vi "construct.vi"(8 "error in (no error)":errorcluster, 9 "configuration name":string, 10 "load config file?":bool=TRUE, 11 "ExperimentControllerDL090130Interval in":refnum<class "ExperimentControllerDL090130Interval.lvclass">) -> (0 "error out":errorcluster, 3 "ExperimentControllerDL090130Interval out":refnum<class "ExperimentControllerDL090130Interval.lvclass">)   [LabVIEW 2010, in "ExperimentControllerDL090130Interval.lvclass"]
uses:
  ExperimentControllerDL090130Interval.lvclass
  GenericExperimentController/GenericExperimentController/GenericExperimentController.lvclass
  ExperimentControllerDL090130Interval.lvclass/ExperimentControllerDL090130Interval.ctl
  Sweep/GenericSweep/GenericSweep/GenericSweep.lvclass
  common/classes/ErrorController/ErrorController/class_data.vi
  common/classes/GenericComponent/GenericComponent/GenericComponent.lvclass
  common/classes/ErrorController/ErrorController/ErrorController.lvclass
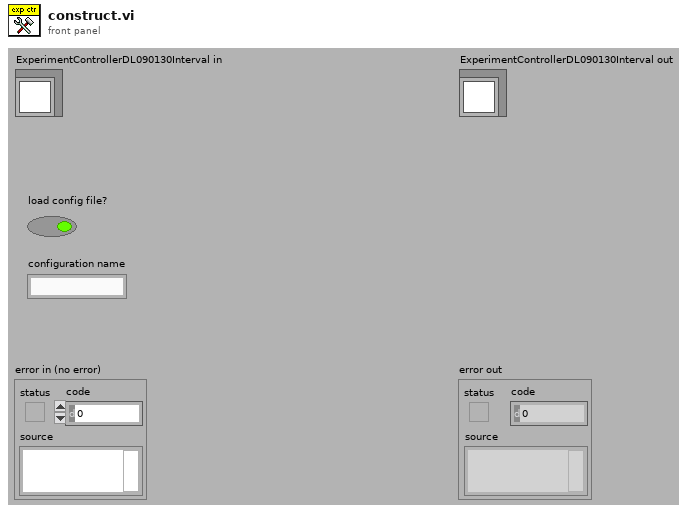
[diagram p1: front panel]
types:
  T1 = typedef "plugin_specification.ctl" = cluster{"class path":string, "configuration":string, "label":string, "settings name":string}
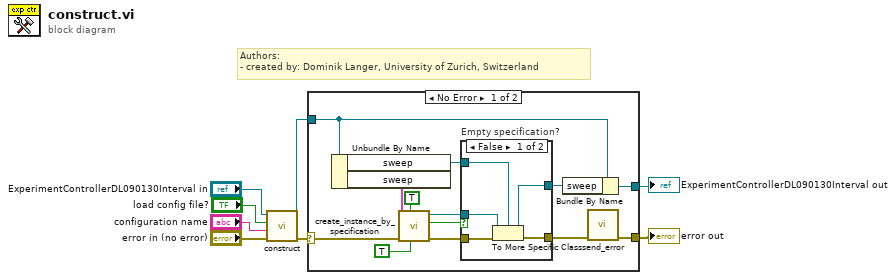
[diagram p0: block diagram]
diagram:
  # "Authors: \n- created by: Dominik Langer, University of Zurich, Switzerland"
  n1 = call-parent "construct.vi"("error in (no error)"="error in (no error)", "configuration name"="configuration name", "load config file?"="load config file?", "GenericPlugin in"="ExperimentControllerDL090130Interval in") -> ("error out"=w4:errorcluster, "GenericPlugin out"=w3:refnum<class "ExperimentControllerDL090130Interval.lvclass">)  [unwired: 6 in]
  n2 = case shown="No Error" w4 {
    selector: w4 -> [w18 w29]
    tunnel: w3 -> [w20 w28]
    tunnel: [w11 w29] -> w2
    tunnel: [w19 w28] -> w1
    frame No Error {
      n3 = Unbundle By Name(w20) -> ("sweep"=w21:refnum<class "GenericSweep.lvclass">, "sweep"=w17:T1)
      n4 = call "create_instance_by_specification.vi"("be tolerant against empty specification?"=TRUE, "call constructor?"=TRUE, "error in (no error)"=w18, "component specification"=w17) -> ("error out"=w16:errorcluster, "empty specification!"=w9:bool, "GenericPlugin out"=w13:refnum<class "GenericComponent.lvclass">)  [unwired: 5 in]
      n5 = case "Empty specification?" shown="False" w9 {
        tunnel: w21 -> [w26 _]
        tunnel: w16 -> [w25 w27]
        tunnel: [w24 _] -> w15
        tunnel: w13 -> [w23 _]
        tunnel: [w22 w27] -> w12
        frame False {
          n6 = To More Specific Class(target class=w26, reference=w23, error in=w25) -> (specific class reference=w24:refnum<class "GenericSweep.lvclass">, error out=w22:errorcluster)
        }
        frame True {
        }
      }
      n7 = Bundle By Name(cluster=w20, "sweep"=w15) -> (w19:refnum<class "ExperimentControllerDL090130Interval.lvclass">)
      n8 = call "send_error.vi"("error in (no error)"=w12) -> ("error out"=w11:errorcluster)  [unwired: 10 in]
    }
    frame Error {
    }
  }
  "error out" <- w2
  "ExperimentControllerDL090130Interval out" <- w1
